vi "PressureYfunction.vi"(9 "Temperature (K)":dbl, 10 "Pressure (mbar)":dbl, 11 "Tube Radius (mm)":dbl=1.2192) -> (3 "Y(r,p,t)":dbl)   [LabVIEW 2025]
doc: "Author: Scott Hannahs <sth@magnet.fsu.edu>\n\nThis software is licensed for use under the “MIT License\"\nCopyright (c) 2025 Scott Hannahs, sth@sth@magnet.sthnet.net\n\nPermission is hereby granted, free of charge, to any person obtaining a copy of this software and associated documentation files (the \"Software\"), to deal in the Software without restriction, including without limitation the rights to use, copy, modify, merge, publish, distribute, sublicense, and/or sell copies of the Software, and to permit persons to whom the Software is furnished to do so, subject to the following conditions: The above copyright notice and this permission notice shall be included in all copies or substantial portions of the Software.\n\nTHE SOFTWARE IS PROVIDED \"AS IS\", WITHOUT WARRANTY OF ANY KIND, EXPRESS OR IMPLIED, INCLUDING BUT NOT LIMITED TO THE WARRANTIES OF MERCHANTABILITY, FITNESS FOR A PARTICULAR PURPOSE AND NONINFRINGEMENT. IN NO EVENT SHALL THE AUTHORS OR COPYRIGHT HOLDERS BE LIABLE FOR ANY CLAIM, DAMAGES OR OTHER LIABILITY, WHETHER IN AN ACTION OF CONTRACT, TORT OR OTHERWISE, ARISING FROM, OUT OF OR IN CONNECTION WITH THE SOFTWARE OR THE USE OR OTHER DEALINGS IN THE SOFTWARE."
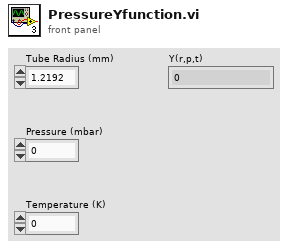
[diagram p1: front panel]
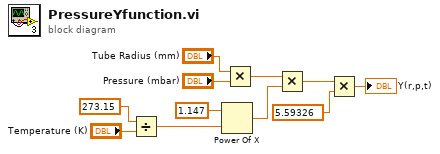
[diagram p0: block diagram]
diagram:
  n1 = Divide(x=273.15, y="Temperature (K)") -> (x/y=w7:dbl)
  n2 = Power Of X(1:w7, 2:1.147 ("y")) -> (0:w5:dbl)
  n3 = Multiply(x="Tube Radius (mm)", y="Pressure (mbar)") -> (x*y=w4:dbl)
  n4 = Multiply(x=w4, y=w5) -> (x*y=w3:dbl)
  n5 = Multiply(x=w3, y=5.59326) -> (x*y=→"Y(r,p,t)":dbl)
